vi "ctn2.vi"(9 "VReff":dbl, 10 "x":dbl, 11 "Numérique":dbl) -> (3 "Numérique 3":dbl)   [LabVIEW 2020]
uses:
  Variables globales outil isospi sans MCU.vi
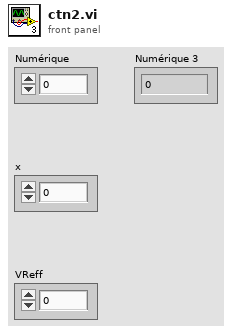
[diagram p1: front panel]
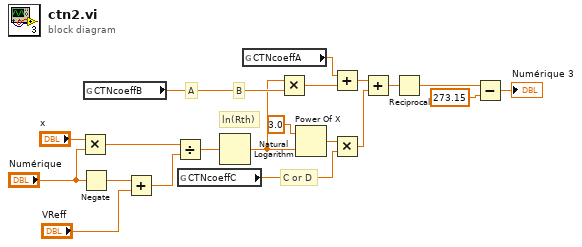
[diagram p0: block diagram]
diagram:
  # "C or D"
  # "B"
  # "ln(Rth)"
  # "A"
  n1 = Multiply(x="x", y="Numérique") -> (x*y=w13:dbl)
  n2 = Negate(x="Numérique") -> (-x=w11:dbl)
  n3 = global read "Variables globales outil isospi sans MCU.vi" "CTNcoeffB"() -> (w19:dbl)
  n4 = Add(x=w11, y="VReff") -> (x+y=w14:dbl)
  n5 = Divide(x=w13, y=w14) -> (x/y=w12:dbl)
  n6 = global read "Variables globales outil isospi sans MCU.vi" "CTNcoeffC"() -> (w20:dbl)
  n7 = Natural Logarithm(1:w12) -> (0:w6:dbl)
  n8 = global read "Variables globales outil isospi sans MCU.vi" "CTNcoeffA"() -> (w18:dbl)
  n9 = Multiply(x=w6, y=w19) -> (x*y=w4:dbl)
  n10 = Power Of X(1:w6, 2:3.0 ("y")) -> (0:w7:dbl)
  n11 = Add(x=w18, y=w4) -> (x+y=w8:dbl)
  n12 = Multiply(x=w7, y=w20) -> (x*y=w9:dbl)
  n13 = Add(x=w8, y=w9) -> (x+y=w10:dbl)
  n14 = Reciprocal(x=w10) -> (1/x=w15:dbl)
  n15 = Subtract(x=w15, y=273.15) -> (x-y=→"Numérique 3":dbl)
